vi "Data Analysis Loop.vi"(8 "Message Queues":T1, 9 "Estimate Notifier In":refnum<notifier>, 10 "DAQ Notifier In":refnum<notifier>, 11 "Estimate Queue In":refnum<queue>) -> (2 "Estimate Notifier Out":refnum<notifier>, 3 "Estimate Queue Out":refnum<queue>)   [LabVIEW 2019]
uses:
  support/Message Queue/All Message Queues.ctl
  support/Message Queue/Message Cluster.ctl
  controls/Components Message Queues.ctl
  EstimateCluster.ctl
  controls/Component Type.ctl
  support/Message Queue/Enqueue Message (Single).vi
  <vilib>/Waveform/WDTOps.llb/WDT Get Final Time Value DBL.vi
  <vilib>/Utility/error.llb/Error Cluster From Error Code.vi
  <vilib>/ErrorRing/Error Ring.xnode
  support/Message Queue/Message Queue.lvlib
panel:
  in  "error in (no error)":errorcluster
  out "error out":errorcluster
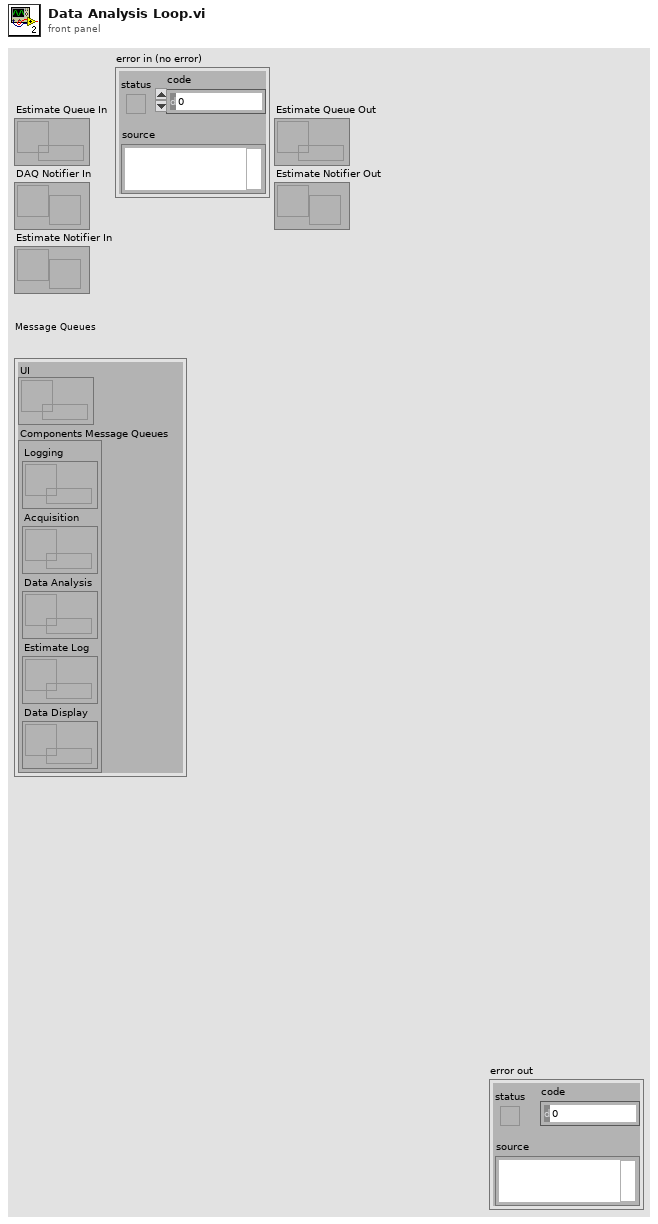
[diagram p1: front panel]
types:
  T1 = typedef "Message Queue.lvlib/All Message Queues.ctl" = cluster{"UI":refnum<queue>, "Components Message Queues":T2}
  T2 = typedef "Message Queue.lvlib/Components Message Queues.ctl" = cluster{"Logging":refnum<queue>, "Acquisition":refnum<queue>, "Data Analysis":refnum<queue>, "Estimate Log":refnum<queue>, "Data Display":refnum<queue>}
  T3 = typedef "EstimateCluster.ctl" = cluster{"Lambda":dbl, "Puissance":dbl, "Rayon":dbl, "Angle":dbl, "dt":dbl, "t0":timestamp}
  T4 = typedef "Component Type.ctl" = enum16{"UI", "Logging", "Acquisition", "Data Analysis", "Estimate", "Data Display"}
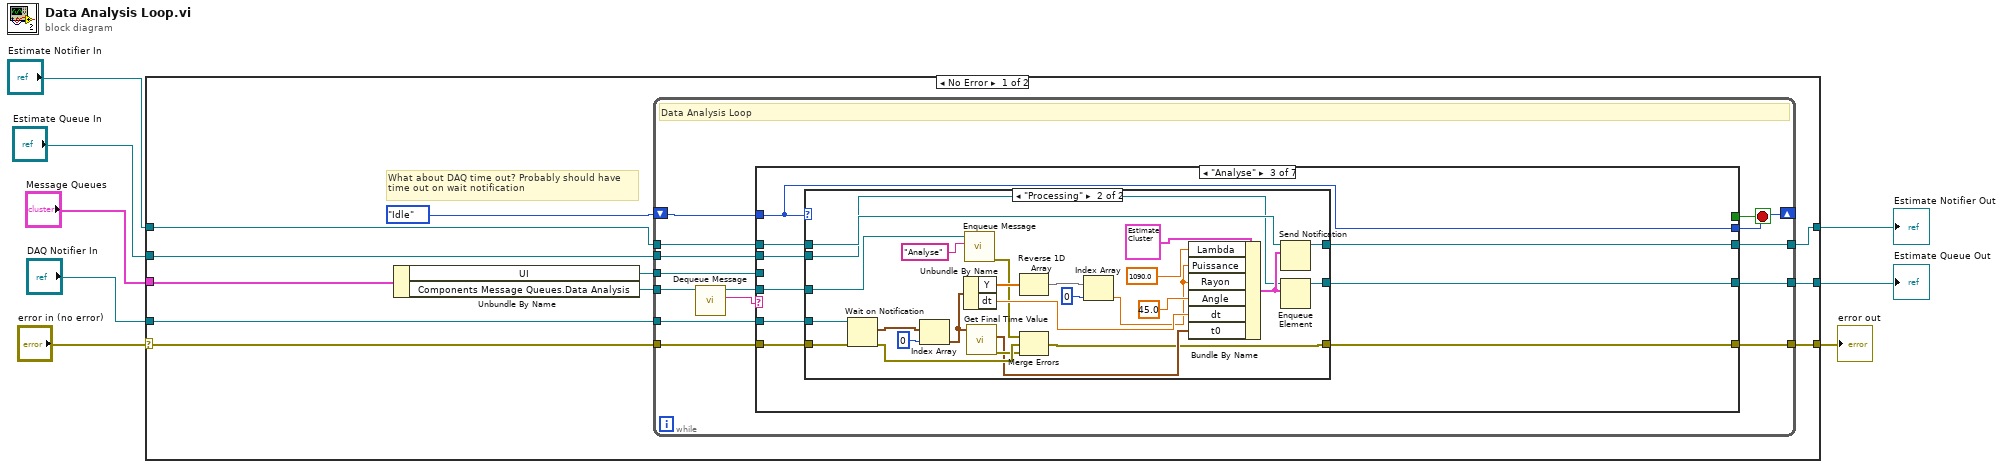
[diagram p0: block diagram]
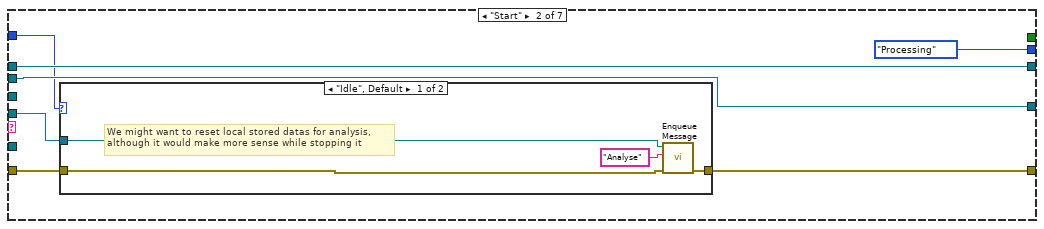
[diagram p3: hidden frame]
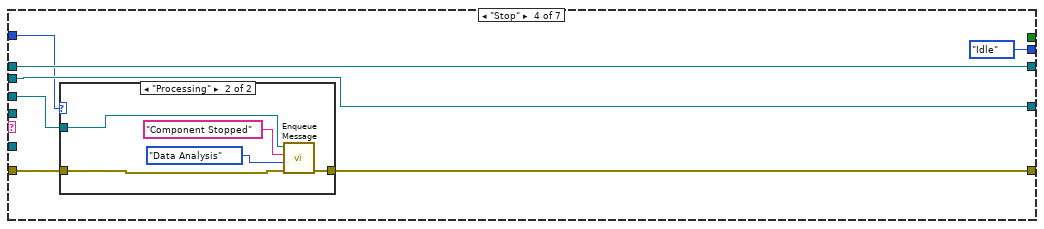
[diagram p6: hidden frame]
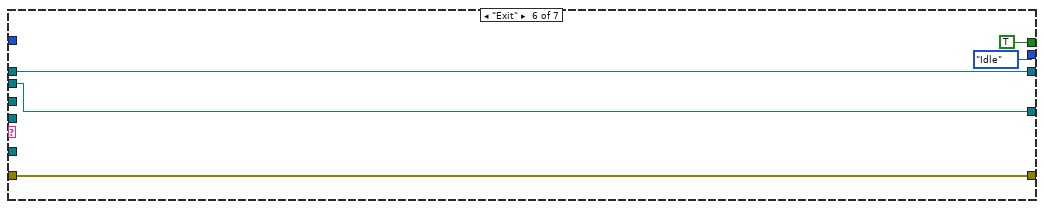
[diagram p9: hidden frame]
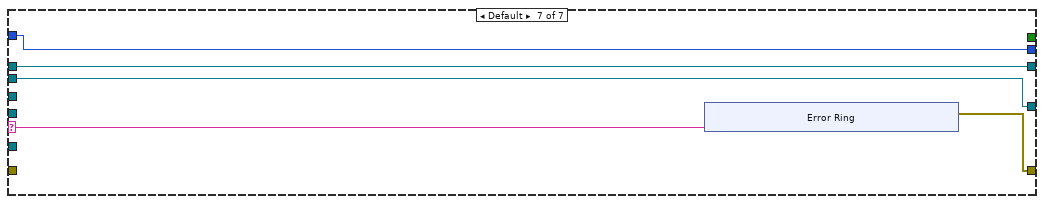
[diagram p10: hidden frame]
diagram:
  n1 = case shown="No Error" "error in (no error)" {
    selector: "error in (no error)" -> [w11 w123]
    tunnel: "DAQ Notifier In" -> [w19 _]
    tunnel: "Message Queues" -> [w14 _]
    tunnel: "Estimate Notifier In" -> [w18 w122]
    tunnel: [w17 w122] -> w5
    tunnel: "Estimate Queue In" -> [w16 w121]
    tunnel: [w15 w121] -> w3
    tunnel: [w10 w123] -> w1
    frame No Error {
      # "What about DAQ time out? Probably should have\ntime out on wait notification"
      n2 = Unbundle By Name(w14) -> ("UI"=w13:refnum<queue>, "Components Message Queues.Data Analysis"=w12:refnum<queue>)
      n3 = while "Data Analysis Loop" {
        tunnel: w19 -> [w33]
        tunnel: w18 -> [w32]
        tunnel: [w31] -> w17
        tunnel: w16 -> [w30]
        tunnel: [w29] -> w15
        tunnel: w13 -> [w22]
        tunnel: w12 -> [w28]
        tunnel: [w27] -> w10
        tunnel: w11 -> [w25]
        shift-right: [w24] -> _
        shift-left: enum16{"Idle", "Processing"}."Idle" -> [w20]
        stop <- w21 stop-if-true
        # "Data Analysis Loop"
        n4 = call "Dequeue Message.vi"("Message Queue"=w28) -> ("Message"=w26:string, "dup Message Queue"=w23:refnum<queue>)  [unwired: 7 in, 2 out]
        n5 = case shown="\"Analyse\"" w26 {
          selector: w26 -> [_ _ _ _ _ _ w110]
          tunnel: w33 -> [_ _ w56 _ _ _ _]
          tunnel: [w37 w38 w55 w87 w103 w108 w111] -> w27
          tunnel: w32 -> [w36 w44 w58 w93 w102 w107 w113]
          tunnel: [w36 w44 w54 w93 w102 w107 w113] -> w31
          tunnel: w30 -> [w35 w43 w57 w92 w101 w106 w112]
          tunnel: [w35 w43 w53 w92 w101 w106 w112] -> w29
          tunnel: w25 -> [w37 w40 w52 w88 w103 w108 _]
          tunnel: w20 -> [w34 w41 w51 w91 w100 _ w109]
          tunnel: [w34 enum16{"Idle", "Processing"}."Processing" w51 enum16{"Idle", "Processing"}."Idle" w100 enum16{"Idle", "Processing"}."Idle" w109] -> w24
          tunnel: w23 -> [_ w39 w50 _ _ _ _]
          tunnel: w22 -> [_ _ _ w89 _ _ _]
          tunnel: [_ _ _ _ _ TRUE _] -> w21
          frame "Initialize" {
          }
          frame "Start" {
            n6 = case shown="\"Idle\", Default" w41 {
              tunnel: w40 -> [w48 w49]
              tunnel: w39 -> [w47 _]
              tunnel: [w46 w49] -> w38
              frame "Idle", Default {
                # "We might want to reset local stored datas for analysis, \nalthough it would make more sense while stopping it"
                n7 = call-poly "Enqueue Message.vi"("error in (no error)"=w48, "Message"="Analyse", "Message Queue"=w47) -> ("error out"=w46:errorcluster)  [unwired: 7 in, 1 out]
              }
              frame "Processing" {
              }
            }
          }
          frame "Analyse" {
            n8 = case shown="\"Processing\"" w51 {
              tunnel: w58 -> [w60 w76]
              tunnel: w57 -> [w59 w72]
              tunnel: w56 -> [_ w71]
              tunnel: [w61 w70] -> w55
              tunnel: [w60 w69] -> w54
              tunnel: [w59 w68] -> w53
              tunnel: w52 -> [w61 w67]
              tunnel: w50 -> [_ w64]
              frame "Idle", Default {
              }
              frame "Processing" {
                n9 = Wait on Notification(notifier=w71, error in (no error)=w67) -> (notification=w79:waveform(dbl)[], error out=w86:errorcluster)  [unwired: 2 in, 2 out]
                n10 = Index Array(array=w79, index=0) -> (element=w83:waveform(dbl))
                n11 = Unbundle By Name(w83) -> ("Y"=w81:dbl[], "dt"=w82:dbl)
                n12 = call-poly "Enqueue Message.vi"("Message"="Analyse", "Message Queue"=w64) -> ("error out"=w65:errorcluster)  [unwired: 8 in, 1 out]
                n13 = call-poly <vilib>:"Get Final Time Value.vi"("waveform in"=w83) -> ("error out"=w85:errorcluster, "tf"=w84:timestamp)  [unwired: 8 in, 1 out]
                n14 = Reverse 1D Array(array=w81) -> (reversed array=w78:dbl[])
                n15 = Merge Errors(w65, w86, w85) -> (w70:errorcluster)
                n16 = Index Array(array=w78, index=0) -> (element=w63:dbl)
                n17 = Bundle By Name(cluster=T3 {"Lambda"=0.0, "Puissance"=0.0, "Rayon"=0.0, "Angle"=0.0, "dt"=0.0, "t0"=timestamp(0 s since 1904-01-01)} ("Estimate Cluster"), "Lambda"=1090.0, "Puissance"=w63, "Rayon"=w63, "Angle"=45.0 ("theta"), "dt"=w82, "t0"=w84) -> (w80:T3)
                n18 = Send Notification(notification=w80, notifier=w76) -> (notifier out=w69:refnum<notifier>)  [unwired: 1 in, 1 out]
                n19 = Enqueue Element(queue=w72, element=w80) -> (queue out=w68:refnum<queue>)  [unwired: 2 in, 2 out]
              }
            }
          }
          frame "Stop" {
            n20 = case shown="\"Processing\"" w91 {
              tunnel: w89 -> [_ w98]
              tunnel: w88 -> [w94 w97]
              tunnel: [w94 w96] -> w87
              frame "Idle", Default {
              }
              frame "Processing" {
                n21 = call-poly "Enqueue Message.vi"("error in (no error)"=w97, "Message Data"=Component_Type."Data Analysis" ("Component Type"), "Message"="Component Stopped", "Message Queue"=w98) -> ("error out"=w96:errorcluster)  [unwired: 6 in, 1 out]
              }
            }
          }
          frame "Reset" {
            # "Nothing to reset yet. Also, I think we should reset it each time we stop."
          }
          frame "Exit" {
          }
          frame Default {
            n22 = xnode "Error Ring"("parameter 0"=w110) -> ("error out"=w111:errorcluster)
          }
        }
      }
    }
    frame Error {
    }
  }
  "error out" <- w1
  "Estimate Notifier Out" <- w5
  "Estimate Queue Out" <- w3
